vi "WinCI Get StaticVI Path.vi"() -> (7 "staticVI path":path)   [LabVIEW 2017, in "NI_SCC_WinCI.lvlib"]
uses:
  <vilib>/SourceControl/Providers/WinCI/NI_SCC_WinCI.lvlib
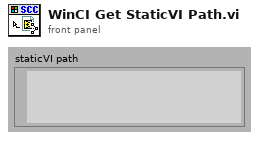
[diagram p1: front panel]
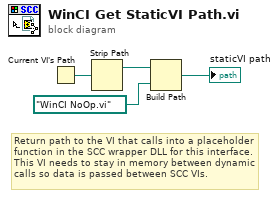
[diagram p0: block diagram]
diagram:
  # "Return path to the VI that calls into a placeholder function in the SCC wrapper DLL for this interface.  This VI needs to stay in memory between dynamic calls so data is passed between SCC VIs."
  n1 = Current VI's Path() -> (path=w4:path)
  n2 = Strip Path(path=w4) -> (stripped path=w3:path)  [unwired: 1 out]
  n3 = Build Path(base path=w3, name or relative path=path "WinCI NoOp.vi") -> (appended path=→"staticVI path":path)
